vi "Inline Write.vi"(8 "error in (no error)":errorcluster, 9 "values":variant[](array[variant]), 10 "keys":string[](array[string]), 11 "uData in":refnum<class "uData.lvclass">) -> (0 "error out":errorcluster, 3 "uData out":refnum<class "uData.lvclass">, 4 "replaced?":bool[](array[boolean]))   [LabVIEW 2021, in "uData.lvlib" / "uData.lvclass"]
doc: "Dynamic dispatch method to perform an inline write operation.\n\n<B>THE \"INLINE\" DYNAMIC DISPATCH METHOD GROUP ARE THE ONLY METHODS THAT ARE ALLOWED TO ACCESS THE OBJECT PRIVATE DATA.</B>\n\nCONVERTED TO INLINE STATIC DISPATCH TO MITIGATE THE PERFORMANCE OVERHEAT HIT REALIZED IN INTIAL TESTING."
uses:
  uData.lvclass
  uData.lvclass/uData.ctl
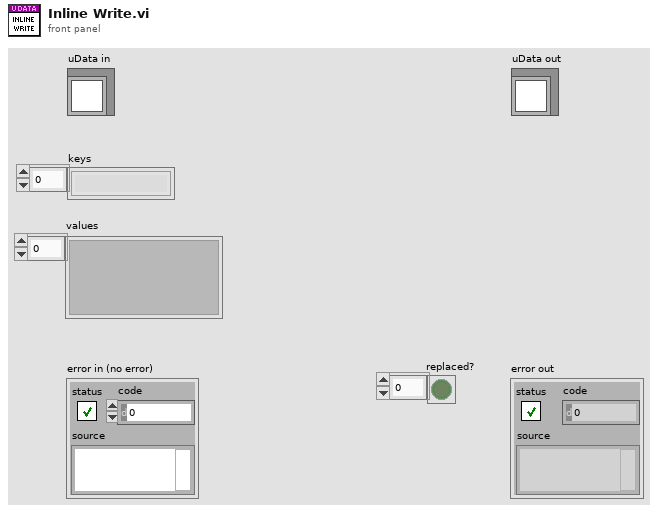
[diagram p1: front panel]
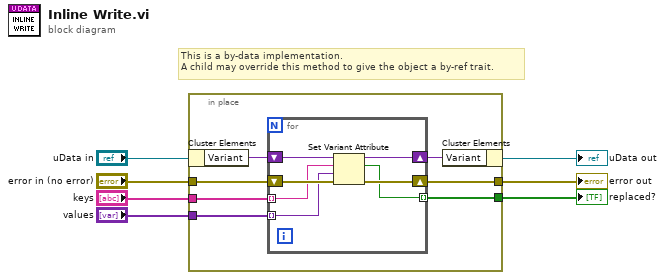
[diagram p0: block diagram]
diagram:
  # "This is a by-data implementation.\nA child may override this method to give the object a by-ref trait."
  n1 = in-place {
    in-place-border: [w12] -> w3
    in-place-border: "error in (no error)" -> [w11]
    in-place-border: [w10] -> w7
    in-place-border: "keys" -> [w8]
    in-place-border: "values" -> [w9]
    n2 = in-place-cluster #1("uData in") -> ("Variant"=w14:variant)
    n3 = for {
      tunnel: [w17] -> w10 mode=indexing
      tunnel: w9 -> [w16] mode=indexing
      tunnel: w8 -> [w15] mode=indexing
      shift-right: [w20] -> w13
      shift-left: w14 -> [w21]
      shift-right: [w19] -> w12
      shift-left: w11 -> [w18]
      n4 = Set Variant Attribute(Variant=w21, name=w15, value=w16, error in=w18) -> (Variant out=w20:variant, replaced=w17:bool, error out=w19:errorcluster)
    }
    n5 = in-place-cluster #1("Variant"=w13) -> (→"uData out":refnum<class "uData.lvclass">)
  }
  "error out" <- w3
  "replaced?" <- w7
